vi "Parallel Operation.vi"(8 "error in (no error)":errorcluster, 9 "Stop Notifier In":refnum<notifier>, 11 "Parallel Operation Actor in":refnum<class "Parallel Operation Actor.lvclass">) -> (0 "error out":errorcluster, 1 "Stop Notifier Out":refnum<notifier>, 3 "Parallel Operation Actor out":refnum<class "Parallel Operation Actor.lvclass">, 4 "Notifier Status":bool)   [LabVIEW 2024, in "Parallel Operation Actor.lvclass"]
uses:
  Parallel Operation Actor.lvclass
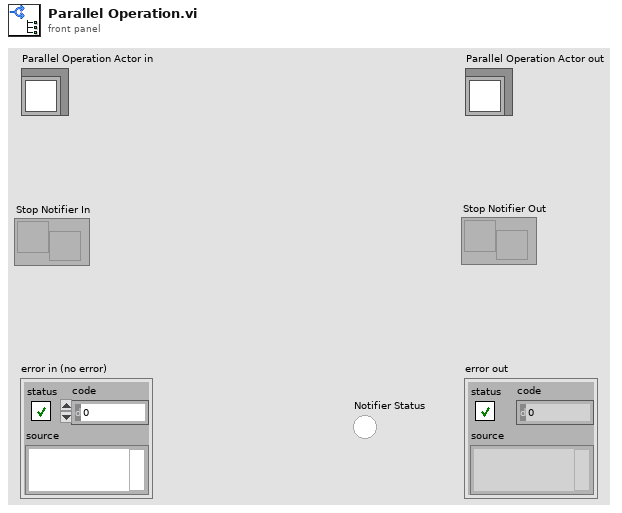
[diagram p1: front panel]
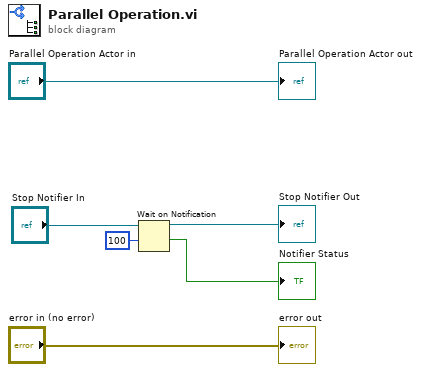
[diagram p0: block diagram]
diagram:
  n1 = Wait on Notification(notifier="Stop Notifier In", timeout in ms (-1)=100) -> (notifier out=→"Stop Notifier Out":refnum<notifier>, timed out?=→"Notifier Status":bool)  [unwired: 2 in, 2 out]
  "error out" <- "error in (no error)"
  "Parallel Operation Actor out" <- "Parallel Operation Actor in"
